vi "Set SubNumber.vi"(8 "error in":errorcluster, 10 "Value":refnum<class "Value.lvclass">, 11 "Object Type in":refnum<class "DOMAIN.lvclass">) -> (0 "error out":errorcluster, 3 "Object Type out":refnum<class "DOMAIN.lvclass">)   [LabVIEW 2024, in "Electronic Datasheet.lvlib" / "DOMAIN.lvclass"]
doc: "Despite for ObjectTypes of Array, SubNumber is not a supported field"
uses:
  DOMAIN.lvclass
  Value/Value.lvclass
  Electronic Datasheet.lvlib
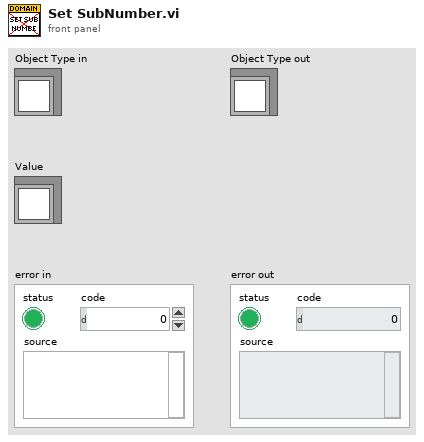
[diagram p1: front panel]
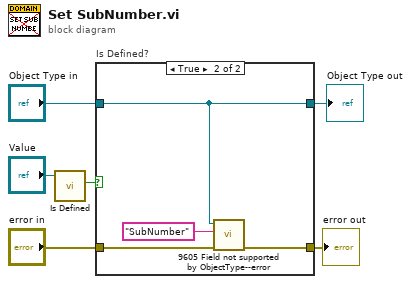
[diagram p0: block diagram]
diagram:
  n1 = call "Is Defined.vi"("Value in"="Value") -> ("Is Defined?"=w5:bool)  [unwired: 9 in, 1 out]
  n2 = case "Is Defined?" shown="True" w5 {
    tunnel: "Object Type in" -> [w7 w10]
    tunnel: [w7 w10] -> w3
    tunnel: "error in" -> [w8 w12]
    tunnel: [w8 w11] -> w1
    frame False {
    }
    frame True {
      n3 = call "9605 Field not supported by ObjectType--error.vi"("error in"=w12, "Field Name"="SubNumber" ("Field name"), "Object Type Base"=w10) -> ("error out"=w11:errorcluster)  [unwired: 8 in]
    }
  }
  "Object Type out" <- w3
  "error out" <- w1
